vi "Get Implementation String.vi"(8 "error in (no error)":errorcluster, 9 "Data In":variant, 10 "Section Name":string, 11 "Configuration File in":refnum<class "Configuration File.lvclass">) -> (0 "error out":errorcluster, 2 "Class Out":refnum<class>, 3 "Configuration File out":refnum<class "Configuration File.lvclass">)   [LabVIEW 2018, in "Configuration File.lvlib" / "Configuration File.lvclass"]
doc: "The VI returns if a class is simulated or not based on the value of the \"Implementation\" string key. The default is blank. This key should exist for every system, since it determines the lvclass object to instantiate in the code.\n\nYou can either wire the section name or the previously read data (to avoid a double read from the file)."
uses:
  Configuration File.lvclass
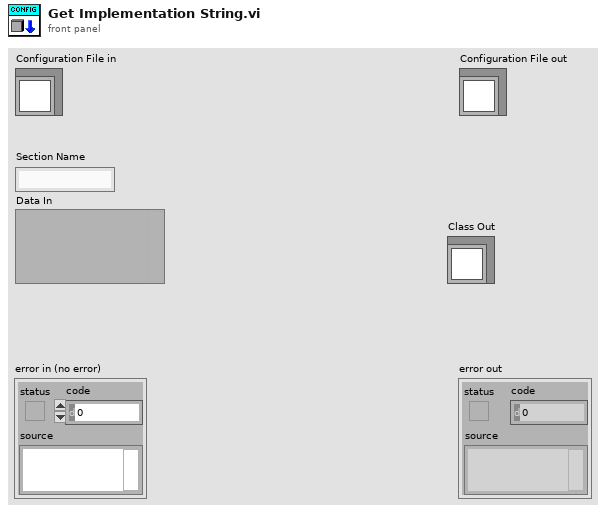
[diagram p1: front panel]
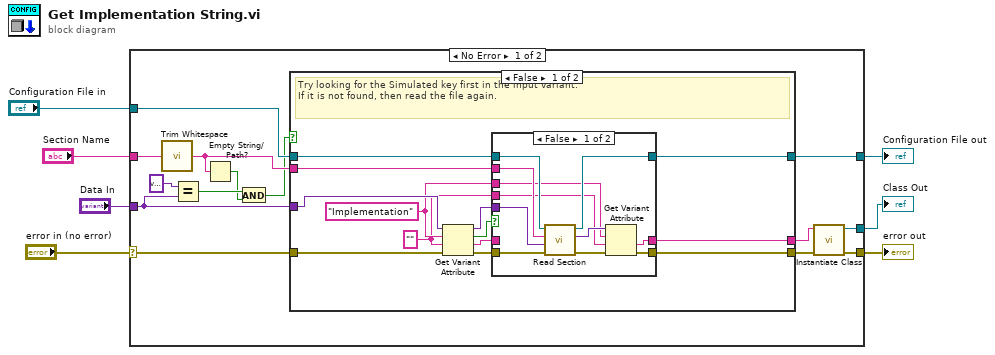
[diagram p0: block diagram]
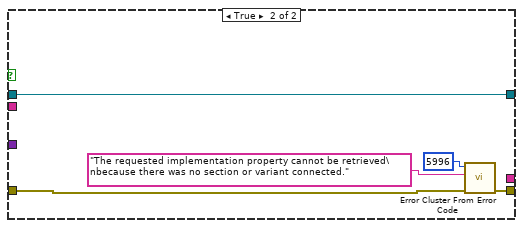
[diagram p3: hidden frame]
diagram:
  n1 = case shown="No Error" "error in (no error)" {
    selector: "error in (no error)" -> [w18 w55]
    tunnel: [w9 w55] -> w6
    tunnel: [w19 w54] -> w4
    tunnel: "Configuration File in" -> [w21 w54]
    tunnel: "Section Name" -> [w20 _]
    tunnel: "Data In" -> [w16 _]
    tunnel: [w10 _] -> w1
    frame No Error {
      n2 = call <vilib>:"Trim Whitespace.vi"("string"=w20) -> ("trimmed string"=w13:string)  [unwired: 1 in]
      n3 = Equal?(x=variant, y=w16) -> (x = y?=w15:bool)
      n4 = Empty String/Path?(string/path=w13) -> (empty?=w14:bool)
      n5 = And(x=w15, y=w14) -> (x .and. y?=w12:bool)
      n6 = case shown="False" w12 {
        tunnel: w21 -> [w34 w53]
        tunnel: w13 -> [w33 _]
        tunnel: [w32 w53] -> w19
        tunnel: [w31 w51] -> w11
        tunnel: [w30 _] -> w8
        tunnel: w16 -> [w29 _]
        tunnel: w18 -> [w27 w52]
        frame False {
          w22 = ""
          w23 = "Implementation" ("name")
          # "Try looking for the Simulated key first in the input variant.\nIf it is not found, then read the file again."
          n7 = Get Variant Attribute(Variant=w29, name=w23, default value (empty Variant)=w22, error in=w27) -> (duplicate Variant=w28:variant, found=w25:bool, value=w24:string, error out=w26:errorcluster)
          n8 = case shown="False" w25 {
            tunnel: w34 -> [w45 w48]
            tunnel: w33 -> [w44 _]
            tunnel: [w43 w48] -> w32
            tunnel: [w40 w46] -> w31
            tunnel: [w39 w47] -> w30
            tunnel: w28 -> [w38 _]
            tunnel: w26 -> [w37 w46]
            tunnel: w24 -> [_ w47]
            tunnel: w23 -> [w36 _]
            tunnel: w22 -> [w35 _]
            frame False {
              n9 = call-dynamic "Read Section.vi"("error in (no error)"=w37, "Data In"=w38, "Section Name"=w44, "Configuration File in"=w45) -> ("error out"=w42:errorcluster, "Data Out"=w41:variant, "Configuration File out"=w43:refnum<class "Configuration File.lvclass">)  [unwired: 4 in, 1 out]
              n10 = Get Variant Attribute(Variant=w41, name=w36, default value (empty Variant)=w35, error in=w42) -> (value=w39:string, error out=w40:errorcluster)  [unwired: 2 out]
            }
            frame True {
            }
          }
        }
        frame True {
          n11 = call <vilib>:"Error Cluster From Error Code.vi"("error in (no error)"=w52, "error message (\"\")"="The requested implementation property cannot be retrieved\nbecause there was no section or variant connected." ("error message (\"\")"), "error code (0)"=5996) -> ("error out"=w51:errorcluster)  [unwired: 6 in]
        }
      }
      n12 = call "Instantiate Class.vi"("error in (no error)"=w11, "String"=w8) -> ("error out"=w9:errorcluster, "LabVIEW Object out"=w10:refnum<class>)  [unwired: 8 in]
    }
    frame Error {
    }
  }
  "error out" <- w6
  "Configuration File out" <- w4
  "Class Out" <- w1
